vi "Single Slow IV v1.3.vi"() -> ()   [LabVIEW 2020]
uses:
  <vilib>/Utility/file.llb/Write Delimited Spreadsheet (DBL).vi
panel:
  in  "stop":bool
  in  "Tab Control 2":enum32{"cRIO plot", "Lockin X", "Lockin Y"}(tab)
  out "cRIO data plot":cluster{"Y":dbl[], "Y":dbl[]}[](graph)=[{"Y"=[0.1, 0.101, 0.10200000000000001, 0.10300000000000001, 0.10400000000000001, 0.10500000000000001, 0.10600000000000001, 0.10700000000000001, 0.10800000000000001, 0.10900000000000001, 0.11, 0.111, 0.112, 0.113, 0.114, 0.115, 0.116, 0.117, 0.11800000000000001, 0.11900000000000001, 0.12000000000000001, 0.12100000000000001, 0.122, 0.123, 0.124, 0.125, 0.126, 0.127, 0.128, 0.129, 0.13, 0.131, 0.132, 0.133, 0.134, 0.135, 0.136, 0.137, 0.138, 0.139, 0.14, 0.14100000000000001, 0.14200000000000002, 0.14300000000000002, 0.14400000000000002, 0.14500000000000002, 0.14600000000000002, 0.14700000000000002, 0.14800000000000002, 0.14900000000000002, 0.15000000000000002, 0.15100000000000002, 0.15200000000000002, 0.153, 0.154, 0.155, 0.156, 0.157, 0.158, 0.159, 0.16, 0.161, 0.162, 0.163, 0.164, 0.165, 0.166, 0.167, 0.168, 0.169, 0.17, 0.171, 0.17200000000000001, 0.173, 0.174, 0.175, 0.176, 0.177, 0.178, 0.179, 0.18, 0.181, 0.182, 0.183, 0.184, 0.185, 0.186, 0.187, 0.188, 0.189, 0.19, 0.191, 0.192, 0.193, 0.194, 0.195, 0.196, 0.197, 0.198, 0.199, 0.2], "Y"=[1.91443115234375e-05, 1.8234204101562503e-05, 1.8079296875e-05, 1.72965576171875e-05, 1.73908447265625e-05, 1.6982641601562502e-05, 1.7475024414062502e-05, 1.7350537109375e-05, 1.80681884765625e-05, 1.8036865234375e-05, 1.8520703124999998e-05, 1.9111669921875e-05, 1.948046875e-05, 1.9645117187500002e-05, 1.95529296875e-05, 1.9983398437500002e-05, 1.99129638671875e-05, 1.99599365234375e-05, 1.8666650390625e-05, 1.8764892578125e-05, 1.78889892578125e-05, 1.7660498046875002e-05, 1.7441210937500002e-05, 1.69652587890625e-05, 1.67341064453125e-05, 1.5950341796875e-05, 1.6491918945312503e-05, 1.61111572265625e-05, 1.6419482421875e-05, 1.6167163085937502e-05, 1.6684667968750002e-05, 1.66596923828125e-05, 1.76610595703125e-05, 1.7373608398437503e-05, 1.7419580078125e-05, 1.7511450195312502e-05, 1.76984619140625e-05, 1.7275e-05, 1.8423168945312502e-05, 1.78859619140625e-05, 1.74806396484375e-05, 1.7222802734375003e-05, 1.6946435546875e-05, 1.5935034179687498e-05, 1.5810864257812502e-05, 1.527841796875e-05, 1.509169921875e-05, 1.4530908203125001e-05, 1.4473876953125001e-05, 1.4885107421875e-05, 1.4928662109374999e-05, 1.5158349609375e-05, 1.5753149414062502e-05, 1.6247314453125003e-05, 1.59515625e-05, 1.62923583984375e-05, 1.64744873046875e-05, 1.65873779296875e-05, 1.7040673828125e-05, 1.65896484375e-05, 1.76021484375e-05, 1.6583422851562498e-05, 1.6492236328125e-05, 1.5975390625e-05, 1.57067138671875e-05, 1.4773681640625001e-05, 1.5178466796875001e-05, 1.4151171875e-05, 1.4718139648437501e-05, 1.453740234375e-05, 1.45205322265625e-05, 1.39417724609375e-05, 1.42656982421875e-05, 1.4501342773437501e-05, 1.4439892578125e-05, 1.47739501953125e-05, 1.47328369140625e-05, 1.46720703125e-05, 1.51514404296875e-05, 1.5362841796875e-05, 1.5647558593750002e-05, 1.612255859375e-05, 1.57461181640625e-05, 1.56584716796875e-05, 1.5264282226562502e-05, 1.4975024414062499e-05, 1.4608837890625003e-05, 1.4593286132812501e-05, 1.44783935546875e-05, 1.40139404296875e-05, 1.36931640625e-05, 1.3610986328125e-05, 1.3888769531250001e-05, 1.35940673828125e-05, 1.35070068359375e-05, 1.3863745117187502e-05, 1.45044677734375e-05, 1.418330078125e-05, 1.45068115234375e-05, 1.4514819335937501e-05, 1.4418505859375001e-05]}, {"Y"=[0.1, 0.101, 0.10200000000000001, 0.10300000000000001, 0.10400000000000001, 0.10500000000000001, 0.10600000000000001, 0.10700000000000001, 0.10800000000000001, 0.10900000000000001, 0.11, 0.111, 0.112, 0.113, 0.114, 0.115, 0.116, 0.117, 0.11800000000000001, 0.11900000000000001, 0.12000000000000001, 0.12100000000000001, 0.122, 0.123, 0.124, 0.125, 0.126, 0.127, 0.128, 0.129, 0.13, 0.131, 0.132, 0.133, 0.134, 0.135, 0.136, 0.137, 0.138, 0.139, 0.14, 0.14100000000000001, 0.14200000000000002, 0.14300000000000002, 0.14400000000000002, 0.14500000000000002, 0.14600000000000002, 0.14700000000000002, 0.14800000000000002, 0.14900000000000002, 0.15000000000000002, 0.15100000000000002, 0.15200000000000002, 0.153, 0.154, 0.155, 0.156, 0.157, 0.158, 0.159, 0.16, 0.161, 0.162, 0.163, 0.164, 0.165, 0.166, 0.167, 0.168, 0.169, 0.17, 0.171, 0.17200000000000001, 0.173, 0.174, 0.175, 0.176, 0.177, 0.178, 0.179, 0.18, 0.181, 0.182, 0.183, 0.184, 0.185, 0.186, 0.187, 0.188, 0.189, 0.19, 0.191, 0.192, 0.193, 0.194, 0.195, 0.196, 0.197, 0.198, 0.199, 0.2], "Y"=[2.07511962890625, 2.0750732421875, 2.074141357421875, 2.075462646484375, 2.075708740234375, 2.074308349609375, 2.074795654296875, 2.07555810546875, 2.0755185546875, 2.07468310546875, 2.074645751953125, 2.074962646484375, 2.0738427734375, 2.074322509765625, 2.07427294921875, 2.074574951171875, 2.075367431640625, 2.07494384765625, 2.074665771484375, 2.074663330078125, 2.07564013671875, 2.074562255859375, 2.074658935546875, 2.074733154296875, 2.07546826171875, 2.074733154296875, 2.074750244140625, 2.07523779296875, 2.07525244140625, 2.074369384765625, 2.075072265625, 2.0747587890625, 2.075584228515625, 2.075943603515625, 2.074529541015625, 2.07461474609375, 2.075067138671875, 2.075061279296875, 2.07536279296875, 2.07553466796875, 2.074748779296875, 2.075227294921875, 2.074936279296875, 2.075556396484375, 2.0753974609375, 2.0758994140625, 2.0761806640625, 2.075328369140625, 2.07436767578125, 2.076673828125, 2.076259765625, 2.075400146484375, 2.075468505859375, 2.075495849609375, 2.076040283203125, 2.0754658203125, 2.075578125, 2.0752451171875, 2.07488134765625, 2.07554736328125, 2.0753955078125, 2.0752822265625, 2.075176513671875, 2.076365478515625, 2.076373046875, 2.076056884765625, 2.07583837890625, 2.075223388671875, 2.0750703125, 2.07514599609375, 2.075769775390625, 2.0751220703125, 2.07619775390625, 2.075202392578125, 2.075671630859375, 2.07513916015625, 2.076079345703125, 2.076094970703125, 2.075864501953125, 2.07488134765625, 2.07613525390625, 2.076350341796875, 2.07625, 2.07523876953125, 2.075680419921875, 2.0746162109375, 2.076003173828125, 2.0753193359375, 2.075281494140625, 2.0755927734375, 2.075462158203125, 2.07468505859375, 2.07553564453125, 2.075280517578125, 2.0758173828125, 2.075341796875, 2.07434033203125, 2.074906005859375, 2.074229248046875, 2.0753671875, 2.0744853515625]}, {"Y"=[0.1, 0.101, 0.10200000000000001, 0.10300000000000001, 0.10400000000000001, 0.10500000000000001, 0.10600000000000001, 0.10700000000000001, 0.10800000000000001, 0.10900000000000001, 0.11, 0.111, 0.112, 0.113, 0.114, 0.115, 0.116, 0.117, 0.11800000000000001, 0.11900000000000001, 0.12000000000000001, 0.12100000000000001, 0.122, 0.123, 0.124, 0.125, 0.126, 0.127, 0.128, 0.129, 0.13, 0.131, 0.132, 0.133, 0.134, 0.135, 0.136, 0.137, 0.138, 0.139, 0.14, 0.14100000000000001, 0.14200000000000002, 0.14300000000000002, 0.14400000000000002, 0.14500000000000002, 0.14600000000000002, 0.14700000000000002, 0.14800000000000002, 0.14900000000000002, 0.15000000000000002, 0.15100000000000002, 0.15200000000000002, 0.153, 0.154, 0.155, 0.156, 0.157, 0.158, 0.159, 0.16, 0.161, 0.162, 0.163, 0.164, 0.165, 0.166, 0.167, 0.168, 0.169, 0.17, 0.171, 0.17200000000000001, 0.173, 0.174, 0.175, 0.176, 0.177, 0.178, 0.179, 0.18, 0.181, 0.182, 0.183, 0.184, 0.185, 0.186, 0.187, 0.188, 0.189, 0.19, 0.191, 0.192, 0.193, 0.194, 0.195, 0.196, 0.197, 0.198, 0.199, 0.2], "Y"=[0.000849365234375, 0.0008095703125, 0.000814453125, 0.00078076171875, 0.000771240234375, 0.000831787109375, 0.000755859375, 0.00079150390625, 0.0008310546875, 0.00079150390625, 0.00074560546875, 0.00078369140625, 0.000753662109375, 0.00079296875, 0.0007275390625, 0.000805419921875, 0.00074658203125, 0.00084375, 0.000741943359375, 0.00080859375, 0.00072705078125, 0.0007802734375, 0.0007021484375, 0.0008046875, 0.000873779296875, 0.000772216796875, 0.0007861328125, 0.000777587890625, 0.00078466796875, 0.00077001953125, 0.000764404296875, 0.0007626953125, 0.000732421875, 0.00077783203125, 0.00079150390625, 0.0007861328125, 0.000770751953125, 0.0008134765625, 0.00080419921875, 0.00079345703125, 0.000803466796875, 0.0007470703125, 0.000757080078125, 0.000783935546875, 0.000799072265625, 0.000781982421875, 0.00076904296875, 0.000742919921875, 0.00082666015625, 0.00078369140625, 0.000858154296875, 0.00076318359375, 0.0006982421875, 0.00071728515625, 0.00077099609375, 0.00078076171875, 0.000766845703125, 0.00076806640625, 0.000752197265625, 0.000720703125, 0.00075830078125, 0.00077099609375, 0.0008076171875, 0.000795166015625, 0.00074365234375, 0.000795166015625, 0.00078125, 0.000791748046875, 0.000809814453125, 0.00074755859375, 0.000774658203125, 0.000756103515625, 0.00083251953125, 0.000758056640625, 0.00082470703125, 0.00077197265625, 0.000834228515625, 0.000770751953125, 0.00077734375, 0.000760009765625, 0.000823974609375, 0.00071533203125, 0.000766357421875, 0.0007548828125, 0.000796630859375, 0.000743408203125, 0.000770751953125, 0.000744384765625, 0.0007314453125, 0.000734130859375, 0.000804443359375, 0.0007275390625, 0.000815673828125, 0.000766357421875, 0.000784912109375, 0.000762451171875, 0.00075, 0.000779296875, 0.000757080078125, 0.000751953125, 0.000764892578125]}, {"Y"=[0.1, 0.101, 0.10200000000000001, 0.10300000000000001, 0.10400000000000001, 0.10500000000000001, 0.10600000000000001, 0.10700000000000001, 0.10800000000000001, 0.10900000000000001, 0.11, 0.111, 0.112, 0.113, 0.114, 0.115, 0.116, 0.117, 0.11800000000000001, 0.11900000000000001, 0.12000000000000001, 0.12100000000000001, 0.122, 0.123, 0.124, 0.125, 0.126, 0.127, 0.128, 0.129, 0.13, 0.131, 0.132, 0.133, 0.134, 0.135, 0.136, 0.137, 0.138, 0.139, 0.14, 0.14100000000000001, 0.14200000000000002, 0.14300000000000002, 0.14400000000000002, 0.14500000000000002, 0.14600000000000002, 0.14700000000000002, 0.14800000000000002, 0.14900000000000002, 0.15000000000000002, 0.15100000000000002, 0.15200000000000002, 0.153, 0.154, 0.155, 0.156, 0.157, 0.158, 0.159, 0.16, 0.161, 0.162, 0.163, 0.164, 0.165, 0.166, 0.167, 0.168, 0.169, 0.17, 0.171, 0.17200000000000001, 0.173, 0.174, 0.175, 0.176, 0.177, 0.178, 0.179, 0.18, 0.181, 0.182, 0.183, 0.184, 0.185, 0.186, 0.187, 0.188, 0.189, 0.19, 0.191, 0.192, 0.193, 0.194, 0.195, 0.196, 0.197, 0.198, 0.199, 0.2], "Y"=[0.00172021484375, 0.001699462890625, 0.001721435546875, 0.001740966796875, 0.001722412109375, 0.001780517578125, 0.001792724609375, 0.00180224609375, 0.001711181640625, 0.00181494140625, 0.001773193359375, 0.001771240234375, 0.00173388671875, 0.001708740234375, 0.00180908203125, 0.001841064453125, 0.001756103515625, 0.00170068359375, 0.00175, 0.001714111328125, 0.001801025390625, 0.001765625, 0.0017099609375, 0.001703857421875, 0.001786865234375, 0.0018046875, 0.001700927734375, 0.001765380859375, 0.001693603515625, 0.00175244140625, 0.0017626953125, 0.0017978515625, 0.001715576171875, 0.001716064453125, 0.00177099609375, 0.00180712890625, 0.001722900390625, 0.001816650390625, 0.001749755859375, 0.00174755859375, 0.001776123046875, 0.00170849609375, 0.00172509765625, 0.001736083984375, 0.00171533203125, 0.001705322265625, 0.001744873046875, 0.001779296875, 0.001696044921875, 0.00173974609375, 0.001815185546875, 0.001720947265625, 0.00178076171875, 0.001763916015625, 0.0017958984375, 0.0017158203125, 0.00179248046875, 0.001754638671875, 0.00173193359375, 0.001706298828125, 0.00173388671875, 0.00166943359375, 0.0017373046875, 0.001741943359375, 0.001747314453125, 0.001755615234375, 0.001791748046875, 0.001772216796875, 0.001737548828125, 0.00176904296875, 0.00175830078125, 0.001655029296875, 0.001769775390625, 0.001682861328125, 0.00176318359375, 0.00177294921875, 0.00177001953125, 0.00178271484375, 0.00175537109375, 0.00174755859375, 0.001724365234375, 0.001774658203125, 0.0017412109375, 0.001767333984375, 0.00175341796875, 0.0017685546875, 0.0017138671875, 0.0017158203125, 0.00172998046875, 0.001653076171875, 0.0017529296875, 0.001751708984375, 0.001750244140625, 0.00172265625, 0.00180859375, 0.00176953125, 0.00177490234375, 0.001733154296875, 0.001750244140625, 0.001706298828125, 0.0017529296875]}]
  out "cRIO Plot 0":string="DC Voltage V"
  out "cRIO Plot 1":string="DC current uA"
  out "cRIO Plot 2":string="dV V"
  out "cRIO Plot 3":string="dI uA"
  out "Lockin X":cluster{"Y":dbl[], "Y":dbl[]}[](graph)=[{"Y"=[0.1, 0.101, 0.10200000000000001, 0.10300000000000001, 0.10400000000000001, 0.10500000000000001, 0.10600000000000001, 0.10700000000000001, 0.10800000000000001, 0.10900000000000001, 0.11, 0.111, 0.112, 0.113, 0.114, 0.115, 0.116, 0.117, 0.11800000000000001, 0.11900000000000001, 0.12000000000000001, 0.12100000000000001, 0.122, 0.123, 0.124, 0.125, 0.126, 0.127, 0.128, 0.129, 0.13, 0.131, 0.132, 0.133, 0.134, 0.135, 0.136, 0.137, 0.138, 0.139, 0.14, 0.14100000000000001, 0.14200000000000002, 0.14300000000000002, 0.14400000000000002, 0.14500000000000002, 0.14600000000000002, 0.14700000000000002, 0.14800000000000002, 0.14900000000000002, 0.15000000000000002, 0.15100000000000002, 0.15200000000000002, 0.153, 0.154, 0.155, 0.156, 0.157, 0.158, 0.159, 0.16, 0.161, 0.162, 0.163, 0.164, 0.165, 0.166, 0.167, 0.168, 0.169, 0.17, 0.171, 0.17200000000000001, 0.173, 0.174, 0.175, 0.176, 0.177, 0.178, 0.179, 0.18, 0.181, 0.182, 0.183, 0.184, 0.185, 0.186, 0.187, 0.188, 0.189, 0.19, 0.191, 0.192, 0.193, 0.194, 0.195, 0.196, 0.197, 0.198, 0.199, 0.2], "Y"=[1.41335, 1.26267, 0.92316, 1.13488, 1.13869, 1.297, 1.30273, 1.3466, 1.35041, 1.09673, 1.13679, 1.0013699999999999, 1.02998, 1.0681200000000002, 0.974659, 0.8926430000000001, 1.33706, 1.05477, 1.02235, 1.29319, 1.03951, 1.3141699999999998, 1.31989, 1.35613, 1.07766, 0.74387, 0.795368, 0.93079, 0.812534, 0.8869210000000001, 1.02235, 1.12153, 1.23788, 1.0585900000000001, 1.02807, 0.928883, 1.13488, 0.9727520000000001, 0.86594, 0.856403, 0.812534, 0.8754770000000001, 1.0604900000000002, 0.963215, 0.957493, 1.00899, 1.08147, 0.8697550000000001, 0.974659, 1.14632, 1.0585900000000001, 0.963215, 0.633243, 0.770573, 1.03761, 0.911716, 0.9594, 1.08529, 1.10436, 1.07766, 0.822071, 0.879291, 1.11008, 1.17493, 1.05477, 0.909809, 0.720982, 0.629429, 0.698093, 0.909809, 0.967029, 0.913624, 0.92316, 0.810627, 0.949863, 1.07384, 1.14823, 1.22262, 1.0662200000000002, 1.01281, 0.8697550000000001, 1.0604900000000002, 0.9594, 0.734333, 0.8316079999999999, 0.835422, 0.8964580000000001, 0.764851, 0.804905, 0.791553, 0.947956, 0.5817450000000001, 0.654224, 0.625614, 0.631336, 0.711445, 0.730518, 0.606541, 0.633243, 0.703815, 0.646595]}, {"Y"=[0.1, 0.101, 0.10200000000000001, 0.10300000000000001, 0.10400000000000001, 0.10500000000000001, 0.10600000000000001, 0.10700000000000001, 0.10800000000000001, 0.10900000000000001, 0.11, 0.111, 0.112, 0.113, 0.114, 0.115, 0.116, 0.117, 0.11800000000000001, 0.11900000000000001, 0.12000000000000001, 0.12100000000000001, 0.122, 0.123, 0.124, 0.125, 0.126, 0.127, 0.128, 0.129, 0.13, 0.131, 0.132, 0.133, 0.134, 0.135, 0.136, 0.137, 0.138, 0.139, 0.14, 0.14100000000000001, 0.14200000000000002, 0.14300000000000002, 0.14400000000000002, 0.14500000000000002, 0.14600000000000002, 0.14700000000000002, 0.14800000000000002, 0.14900000000000002, 0.15000000000000002, 0.15100000000000002, 0.15200000000000002, 0.153, 0.154, 0.155, 0.156, 0.157, 0.158, 0.159, 0.16, 0.161, 0.162, 0.163, 0.164, 0.165, 0.166, 0.167, 0.168, 0.169, 0.17, 0.171, 0.17200000000000001, 0.173, 0.174, 0.175, 0.176, 0.177, 0.178, 0.179, 0.18, 0.181, 0.182, 0.183, 0.184, 0.185, 0.186, 0.187, 0.188, 0.189, 0.19, 0.191, 0.192, 0.193, 0.194, 0.195, 0.196, 0.197, 0.198, 0.199, 0.2], "Y"=[0.755314, 0.915531, 0.9594, 0.967029, 0.9727520000000001, 0.970844, 0.970844, 0.974659, 0.970844, 0.974659, 0.974659, 0.974659, 0.9727520000000001, 0.9727520000000001, 0.974659, 0.970844, 0.9727520000000001, 0.9765699999999999, 0.9765699999999999, 0.9765699999999999, 0.974659, 0.9765699999999999, 0.9803850000000001, 0.9765699999999999, 0.9765699999999999, 0.974659, 0.9727520000000001, 0.9727520000000001, 0.9727520000000001, 0.9765699999999999, 0.974659, 0.9784769999999999, 0.9784769999999999, 0.974659, 0.968937, 0.967029, 0.970844, 0.9765699999999999, 0.9765699999999999, 0.974659, 0.9727520000000001, 0.9727520000000001, 0.9765699999999999, 0.9765699999999999, 0.9765699999999999, 0.974659, 0.9765699999999999, 0.9765699999999999, 0.9765699999999999, 0.9727520000000001, 0.9727520000000001, 0.9765699999999999, 0.9803850000000001, 0.982292, 0.9784769999999999, 0.9784769999999999, 0.974659, 0.974659, 0.9765699999999999, 0.974659, 0.974659, 0.9727520000000001, 0.9765699999999999, 0.9784769999999999, 0.984199, 0.982292, 0.9765699999999999, 0.9765699999999999, 0.974659, 0.974659, 0.9765699999999999, 0.9765699999999999, 0.9765699999999999, 0.9784769999999999, 0.9765699999999999, 0.9765699999999999, 0.9765699999999999, 0.9765699999999999, 0.974659, 0.9765699999999999, 0.9765699999999999, 0.9765699999999999, 0.970844, 0.970844, 0.9765699999999999, 0.9727520000000001, 0.970844, 0.968937, 0.9727520000000001, 0.9765699999999999, 0.9765699999999999, 0.9784769999999999, 0.9765699999999999, 0.9765699999999999, 0.9765699999999999, 0.9765699999999999, 0.9727520000000001, 0.968937, 0.968937, 0.967029, 0.9727520000000001]}, {"Y"=[0.1, 0.101, 0.10200000000000001, 0.10300000000000001, 0.10400000000000001, 0.10500000000000001, 0.10600000000000001, 0.10700000000000001, 0.10800000000000001, 0.10900000000000001, 0.11, 0.111, 0.112, 0.113, 0.114, 0.115, 0.116, 0.117, 0.11800000000000001, 0.11900000000000001, 0.12000000000000001, 0.12100000000000001, 0.122, 0.123, 0.124, 0.125, 0.126, 0.127, 0.128, 0.129, 0.13, 0.131, 0.132, 0.133, 0.134, 0.135, 0.136, 0.137, 0.138, 0.139, 0.14, 0.14100000000000001, 0.14200000000000002, 0.14300000000000002, 0.14400000000000002, 0.14500000000000002, 0.14600000000000002, 0.14700000000000002, 0.14800000000000002, 0.14900000000000002, 0.15000000000000002, 0.15100000000000002, 0.15200000000000002, 0.153, 0.154, 0.155, 0.156, 0.157, 0.158, 0.159, 0.16, 0.161, 0.162, 0.163, 0.164, 0.165, 0.166, 0.167, 0.168, 0.169, 0.17, 0.171, 0.17200000000000001, 0.173, 0.174, 0.175, 0.176, 0.177, 0.178, 0.179, 0.18, 0.181, 0.182, 0.183, 0.184, 0.185, 0.186, 0.187, 0.188, 0.189, 0.19, 0.191, 0.192, 0.193, 0.194, 0.195, 0.196, 0.197, 0.198, 0.199, 0.2], "Y"=[0.0, 0.0, 0.0, 0.0, 0.0, 0.0, 0.0, 0.0, 0.0, 0.0, 0.0, 0.0, 0.0, 0.0, 0.0, 0.0, 0.0, 0.0, 0.0, 0.0, 0.0, 0.0, 0.0, 0.0, 0.0, 0.0, 0.0, 0.0, 0.0, 0.0, 0.0, 0.0, 0.0, 0.0, 0.0, 0.0, 0.0, 0.0, 0.0, 0.0, 0.0, 0.0, 0.0, 0.0, 0.0, 0.0, 0.0, 0.0, 0.0, 0.0, 0.0, 0.0, 0.0, 0.0, 0.0, 0.0, 0.0, 0.0, 0.0, 0.0, 0.0, 0.0, 0.0, 0.0, 0.0, 0.0, 0.0, 0.0, 0.0, 0.0, 0.0, 0.0, 0.0, 0.0, 0.0, 0.0, 0.0, 0.0, 0.0, 0.0, 0.0, 0.0, 0.0, 0.0, 0.0, 0.0, 0.0, 0.0, 0.0, 0.0, 0.0, 0.0, 0.0, 0.0, 0.0, 0.0, 0.0, 0.0, 0.0, 0.0, 0.0]}, {"Y"=[0.1, 0.101, 0.10200000000000001, 0.10300000000000001, 0.10400000000000001, 0.10500000000000001, 0.10600000000000001, 0.10700000000000001, 0.10800000000000001, 0.10900000000000001, 0.11, 0.111, 0.112, 0.113, 0.114, 0.115, 0.116, 0.117, 0.11800000000000001, 0.11900000000000001, 0.12000000000000001, 0.12100000000000001, 0.122, 0.123, 0.124, 0.125, 0.126, 0.127, 0.128, 0.129, 0.13, 0.131, 0.132, 0.133, 0.134, 0.135, 0.136, 0.137, 0.138, 0.139, 0.14, 0.14100000000000001, 0.14200000000000002, 0.14300000000000002, 0.14400000000000002, 0.14500000000000002, 0.14600000000000002, 0.14700000000000002, 0.14800000000000002, 0.14900000000000002, 0.15000000000000002, 0.15100000000000002, 0.15200000000000002, 0.153, 0.154, 0.155, 0.156, 0.157, 0.158, 0.159, 0.16, 0.161, 0.162, 0.163, 0.164, 0.165, 0.166, 0.167, 0.168, 0.169, 0.17, 0.171, 0.17200000000000001, 0.173, 0.174, 0.175, 0.176, 0.177, 0.178, 0.179, 0.18, 0.181, 0.182, 0.183, 0.184, 0.185, 0.186, 0.187, 0.188, 0.189, 0.19, 0.191, 0.192, 0.193, 0.194, 0.195, 0.196, 0.197, 0.198, 0.199, 0.2], "Y"=[0.0, 0.0, 0.0, 0.0, 0.0, 0.0, 0.0, 0.0, 0.0, 0.0, 0.0, 0.0, 0.0, 0.0, 0.0, 0.0, 0.0, 0.0, 0.0, 0.0, 0.0, 0.0, 0.0, 0.0, 0.0, 0.0, 0.0, 0.0, 0.0, 0.0, 0.0, 0.0, 0.0, 0.0, 0.0, 0.0, 0.0, 0.0, 0.0, 0.0, 0.0, 0.0, 0.0, 0.0, 0.0, 0.0, 0.0, 0.0, 0.0, 0.0, 0.0, 0.0, 0.0, 0.0, 0.0, 0.0, 0.0, 0.0, 0.0, 0.0, 0.0, 0.0, 0.0, 0.0, 0.0, 0.0, 0.0, 0.0, 0.0, 0.0, 0.0, 0.0, 0.0, 0.0, 0.0, 0.0, 0.0, 0.0, 0.0, 0.0, 0.0, 0.0, 0.0, 0.0, 0.0, 0.0, 0.0, 0.0, 0.0, 0.0, 0.0, 0.0, 0.0, 0.0, 0.0, 0.0, 0.0, 0.0, 0.0, 0.0, 0.0]}]
  out "Lockin Y":cluster{"Y":dbl[], "Y":dbl[]}[](graph)=[{"Y"=[0.1, 0.101, 0.10200000000000001, 0.10300000000000001, 0.10400000000000001, 0.10500000000000001, 0.10600000000000001, 0.10700000000000001, 0.10800000000000001, 0.10900000000000001, 0.11, 0.111, 0.112, 0.113, 0.114, 0.115, 0.116, 0.117, 0.11800000000000001, 0.11900000000000001, 0.12000000000000001, 0.12100000000000001, 0.122, 0.123, 0.124, 0.125, 0.126, 0.127, 0.128, 0.129, 0.13, 0.131, 0.132, 0.133, 0.134, 0.135, 0.136, 0.137, 0.138, 0.139, 0.14, 0.14100000000000001, 0.14200000000000002, 0.14300000000000002, 0.14400000000000002, 0.14500000000000002, 0.14600000000000002, 0.14700000000000002, 0.14800000000000002, 0.14900000000000002, 0.15000000000000002, 0.15100000000000002, 0.15200000000000002, 0.153, 0.154, 0.155, 0.156, 0.157, 0.158, 0.159, 0.16, 0.161, 0.162, 0.163, 0.164, 0.165, 0.166, 0.167, 0.168, 0.169, 0.17, 0.171, 0.17200000000000001, 0.173, 0.174, 0.175, 0.176, 0.177, 0.178, 0.179, 0.18, 0.181, 0.182, 0.183, 0.184, 0.185, 0.186, 0.187, 0.188, 0.189, 0.19, 0.191, 0.192, 0.193, 0.194, 0.195, 0.196, 0.197, 0.198, 0.199, 0.2], "Y"=[-0.349047, -0.234605, -0.135423, -0.265123, -0.20408700000000002, -0.144959, -0.106812, 0.0953679, -0.0953679, -0.5397829999999999, -0.608448, -0.364305, -0.33951000000000003, -0.38337899999999997, -0.261309, -0.08010909999999999, 0.0114442, -0.0877385, 0.164033, 0.0381472, -0.034332499999999995, -0.265123, -0.0915532, -0.026703, -0.0953679, -0.06866499999999999, -0.17357, -0.27275299999999997, -0.270845, -0.17357, -0.0762944, -0.23842000000000002, -0.253679, -0.175477, -0.316622, 0.0839238, -0.0743871, -0.278475, -0.164033, -0.23079, -0.305178, -0.33188100000000004, -0.234605, -0.16975500000000002, -0.278475, -0.146867, -0.186921, -0.389101, -0.411989, -0.349047, -0.20790199999999998, -0.026703, -0.26893799999999995, -0.13732999999999998, 0.0743871, -0.020981, -0.0667577, -0.156404, -0.167848, 0.110627, 0.400545, 0.16975500000000002, -0.118256, -0.034332499999999995, 0.108719, 0.167848, 0.127793, 0.07247970000000001, 0.062943, 0.0915532, 0.0839238, -0.0171663, 0.0572207, 0.053406, -0.23079, -0.16594, -0.307085, -0.379564, -0.118256, -0.125886, -0.183106, -0.125886, 0.0419619, -0.0667577, -0.055313299999999996, -0.059128, 0.034332499999999995, 0.0610356, -0.116349, -0.144959, -0.24605, -0.240327, -0.318529, -0.352861, -0.356676, -0.110627, -0.102997, -0.0972752, 0.20408700000000002, 0.144959, 0.20218]}, {"Y"=[0.1, 0.101, 0.10200000000000001, 0.10300000000000001, 0.10400000000000001, 0.10500000000000001, 0.10600000000000001, 0.10700000000000001, 0.10800000000000001, 0.10900000000000001, 0.11, 0.111, 0.112, 0.113, 0.114, 0.115, 0.116, 0.117, 0.11800000000000001, 0.11900000000000001, 0.12000000000000001, 0.12100000000000001, 0.122, 0.123, 0.124, 0.125, 0.126, 0.127, 0.128, 0.129, 0.13, 0.131, 0.132, 0.133, 0.134, 0.135, 0.136, 0.137, 0.138, 0.139, 0.14, 0.14100000000000001, 0.14200000000000002, 0.14300000000000002, 0.14400000000000002, 0.14500000000000002, 0.14600000000000002, 0.14700000000000002, 0.14800000000000002, 0.14900000000000002, 0.15000000000000002, 0.15100000000000002, 0.15200000000000002, 0.153, 0.154, 0.155, 0.156, 0.157, 0.158, 0.159, 0.16, 0.161, 0.162, 0.163, 0.164, 0.165, 0.166, 0.167, 0.168, 0.169, 0.17, 0.171, 0.17200000000000001, 0.173, 0.174, 0.175, 0.176, 0.177, 0.178, 0.179, 0.18, 0.181, 0.182, 0.183, 0.184, 0.185, 0.186, 0.187, 0.188, 0.189, 0.19, 0.191, 0.192, 0.193, 0.194, 0.195, 0.196, 0.197, 0.198, 0.199, 0.2], "Y"=[-0.20790199999999998, -0.114441, -0.0915532, -0.0858312, -0.08010909999999999, -0.0820165, -0.0858312, -0.0839238, -0.0858312, -0.0858312, -0.0858312, -0.0896459, -0.0839238, -0.0858312, -0.0858312, -0.0877385, -0.0877385, -0.0839238, -0.0820165, -0.0858312, -0.0820165, -0.0839238, -0.0858312, -0.0896459, -0.0915532, -0.0877385, -0.0839238, -0.0877385, -0.0877385, -0.0820165, -0.0839238, -0.0820165, -0.0839238, -0.0839238, -0.08010909999999999, -0.0839238, -0.0820165, -0.0877385, -0.0839238, -0.0858312, -0.0858312, -0.0820165, -0.0820165, -0.08010909999999999, -0.0877385, -0.0915532, -0.0934605, -0.0877385, -0.0820165, -0.08010909999999999, -0.08010909999999999, -0.0858312, -0.0820165, -0.0820165, -0.0896459, -0.0877385, -0.0877385, -0.0858312, -0.0839238, -0.08010909999999999, -0.0858312, -0.0839238, -0.08010909999999999, -0.08010909999999999, -0.0839238, -0.08010909999999999, -0.0839238, -0.0877385, -0.0915532, -0.0858312, -0.0839238, -0.0858312, -0.0896459, -0.0915532, -0.0877385, -0.0839238, -0.08010909999999999, -0.08010909999999999, -0.0820165, -0.0820165, -0.0839238, -0.08010909999999999, -0.0839238, -0.0858312, -0.0858312, -0.0915532, -0.0896459, -0.0820165, -0.07820179999999999, -0.08010909999999999, -0.0820165, -0.08010909999999999, -0.0762944, -0.0820165, -0.0820165, -0.0858312, -0.0820165, -0.08010909999999999, -0.0858312, -0.0896459, -0.0877385]}, {"Y"=[0.1, 0.101, 0.10200000000000001, 0.10300000000000001, 0.10400000000000001, 0.10500000000000001, 0.10600000000000001, 0.10700000000000001, 0.10800000000000001, 0.10900000000000001, 0.11, 0.111, 0.112, 0.113, 0.114, 0.115, 0.116, 0.117, 0.11800000000000001, 0.11900000000000001, 0.12000000000000001, 0.12100000000000001, 0.122, 0.123, 0.124, 0.125, 0.126, 0.127, 0.128, 0.129, 0.13, 0.131, 0.132, 0.133, 0.134, 0.135, 0.136, 0.137, 0.138, 0.139, 0.14, 0.14100000000000001, 0.14200000000000002, 0.14300000000000002, 0.14400000000000002, 0.14500000000000002, 0.14600000000000002, 0.14700000000000002, 0.14800000000000002, 0.14900000000000002, 0.15000000000000002, 0.15100000000000002, 0.15200000000000002, 0.153, 0.154, 0.155, 0.156, 0.157, 0.158, 0.159, 0.16, 0.161, 0.162, 0.163, 0.164, 0.165, 0.166, 0.167, 0.168, 0.169, 0.17, 0.171, 0.17200000000000001, 0.173, 0.174, 0.175, 0.176, 0.177, 0.178, 0.179, 0.18, 0.181, 0.182, 0.183, 0.184, 0.185, 0.186, 0.187, 0.188, 0.189, 0.19, 0.191, 0.192, 0.193, 0.194, 0.195, 0.196, 0.197, 0.198, 0.199, 0.2], "Y"=[0.0, 0.0, 0.0, 0.0, 0.0, 0.0, 0.0, 0.0, 0.0, 0.0, 0.0, 0.0, 0.0, 0.0, 0.0, 0.0, 0.0, 0.0, 0.0, 0.0, 0.0, 0.0, 0.0, 0.0, 0.0, 0.0, 0.0, 0.0, 0.0, 0.0, 0.0, 0.0, 0.0, 0.0, 0.0, 0.0, 0.0, 0.0, 0.0, 0.0, 0.0, 0.0, 0.0, 0.0, 0.0, 0.0, 0.0, 0.0, 0.0, 0.0, 0.0, 0.0, 0.0, 0.0, 0.0, 0.0, 0.0, 0.0, 0.0, 0.0, 0.0, 0.0, 0.0, 0.0, 0.0, 0.0, 0.0, 0.0, 0.0, 0.0, 0.0, 0.0, 0.0, 0.0, 0.0, 0.0, 0.0, 0.0, 0.0, 0.0, 0.0, 0.0, 0.0, 0.0, 0.0, 0.0, 0.0, 0.0, 0.0, 0.0, 0.0, 0.0, 0.0, 0.0, 0.0, 0.0, 0.0, 0.0, 0.0, 0.0, 0.0]}, {"Y"=[0.1, 0.101, 0.10200000000000001, 0.10300000000000001, 0.10400000000000001, 0.10500000000000001, 0.10600000000000001, 0.10700000000000001, 0.10800000000000001, 0.10900000000000001, 0.11, 0.111, 0.112, 0.113, 0.114, 0.115, 0.116, 0.117, 0.11800000000000001, 0.11900000000000001, 0.12000000000000001, 0.12100000000000001, 0.122, 0.123, 0.124, 0.125, 0.126, 0.127, 0.128, 0.129, 0.13, 0.131, 0.132, 0.133, 0.134, 0.135, 0.136, 0.137, 0.138, 0.139, 0.14, 0.14100000000000001, 0.14200000000000002, 0.14300000000000002, 0.14400000000000002, 0.14500000000000002, 0.14600000000000002, 0.14700000000000002, 0.14800000000000002, 0.14900000000000002, 0.15000000000000002, 0.15100000000000002, 0.15200000000000002, 0.153, 0.154, 0.155, 0.156, 0.157, 0.158, 0.159, 0.16, 0.161, 0.162, 0.163, 0.164, 0.165, 0.166, 0.167, 0.168, 0.169, 0.17, 0.171, 0.17200000000000001, 0.173, 0.174, 0.175, 0.176, 0.177, 0.178, 0.179, 0.18, 0.181, 0.182, 0.183, 0.184, 0.185, 0.186, 0.187, 0.188, 0.189, 0.19, 0.191, 0.192, 0.193, 0.194, 0.195, 0.196, 0.197, 0.198, 0.199, 0.2], "Y"=[0.0, 0.0, 0.0, 0.0, 0.0, 0.0, 0.0, 0.0, 0.0, 0.0, 0.0, 0.0, 0.0, 0.0, 0.0, 0.0, 0.0, 0.0, 0.0, 0.0, 0.0, 0.0, 0.0, 0.0, 0.0, 0.0, 0.0, 0.0, 0.0, 0.0, 0.0, 0.0, 0.0, 0.0, 0.0, 0.0, 0.0, 0.0, 0.0, 0.0, 0.0, 0.0, 0.0, 0.0, 0.0, 0.0, 0.0, 0.0, 0.0, 0.0, 0.0, 0.0, 0.0, 0.0, 0.0, 0.0, 0.0, 0.0, 0.0, 0.0, 0.0, 0.0, 0.0, 0.0, 0.0, 0.0, 0.0, 0.0, 0.0, 0.0, 0.0, 0.0, 0.0, 0.0, 0.0, 0.0, 0.0, 0.0, 0.0, 0.0, 0.0, 0.0, 0.0, 0.0, 0.0, 0.0, 0.0, 0.0, 0.0, 0.0, 0.0, 0.0, 0.0, 0.0, 0.0, 0.0, 0.0, 0.0, 0.0, 0.0, 0.0]}]
  in  "Tab Control":enum32{"cRIO", "variable", "Lockin", "Status"}(tab)=enum."variable"
  in  "cRIO Chan 0":bool=TRUE
  in  "cRIO IP":string="//172.22.11.2"
  in  "Reading Average times":i32=1000
  in  "read cRIO":bool=TRUE
  in  "Scale factor3":dbl=1.0
  in  "Channel name 3":string(combo)="dI uA"
  in  "cRIO Chan 3":bool
  in  "Scale factor2":dbl=1.0
  in  "Channel name 2":string(combo)="dV V"
  in  "cRIO Chan 2":bool
  in  "Scale factor1":dbl=1.0
  in  "Channel name 1":string(combo)="DC current uA"
  in  "cRIO Chan 1":bool=TRUE
  in  "Scale factor0":dbl=0.0001
  in  "Channel name 0":string(combo)="DC Voltage V"
  out "Unit":string="mT"
  in  "Tab for variable":enum32{"Current", "Magnetic field"}(tab)=enum."Magnetic field"
  in  "Delay Time s":dbl=1.5 caption="Delay Time (s)"
  in  "AO Channel":string(combo)="AO0"
  in  "current output Scale factor":dbl=1.0
  in  "Fixed current uA":dbl=2.1
  in  "Scale factor":dbl=1.0
  in  "Field Rate mT per sec":dbl=0.1 format="%#_13g"
  in  "Magnet Device Select":string(combo)="NI DAQ Controlled V to I source"
  in  "Start":dbl=0.1
  in  "Range":dbl=0.1
  in  "Step":dbl=0.001
  in  "Ramp type":string(combo)="Range"
  in  "Ramp up first T":bool=TRUE
  in  "Lockin address 4":string
  in  "Lockin address 3":string
  in  "Lockin address 2":string="GPIB0::9::INSTR"
  in  "Lockin address 1":string="GPIB0::8::INSTR"
  in  "Lockin 4":bool
  in  "Lockin 3":bool
  in  "Lockin 2":bool=TRUE
  in  "Lockin 1":bool=TRUE
  in  "Use Lockin":bool=TRUE
  in  "Lockin Chan name 4":string(combo)="None"
  in  "Lockin Chan name 3":string(combo)="None"
  in  "Lockin Chan name 2":string(combo)="Current mV"
  in  "Lockin Chan name 1":string(combo)="Voltage mV"
  in  "Lockin and field and temperature status":string="Data File time stamp 20210723-212111\nTemperature Chan1 1.218210, Chan2 0.050013\nmagnetic field InfmT\nLockin status\n#Device channel name Voltage mV#Device \u0000\u0000\u0000\u000fGPIB0::8::INSTR\n #PHASE=0\n #REF=1\n #FREQ=17\n #INPUT=0\n #SENS=22\n #TIMECONST=10\n #VOLTAGE=0.1\n#Device channel name Current mV#Device \u0000\u0000\u0000\u000fGPIB0::9::INSTR\n #PHASE=0\n #REF=0\n #FREQ=16.9997\n #INPUT=0\n #SENS=22\n #TIMECONST=10\n #VOLTAGE=0.004\n"
  in  "Temp Device":string(combo)="Elsa"
  in  "Temp Chan1":string="T5"
  in  "Temp Chan2":string="T8"
  in  "Magnetic field read device":string(combo)="Elsa Magnet"
  in  "Record Field":bool
  in  "Contour plot folder":path=path "C:/Users/gyue/Desktop/Data folder 20210720"
  out "error out":errorcluster
  # "Voltage x factor=actual"
  # "Voltage x factor=uA"
  # "Voltage x factor=uA"
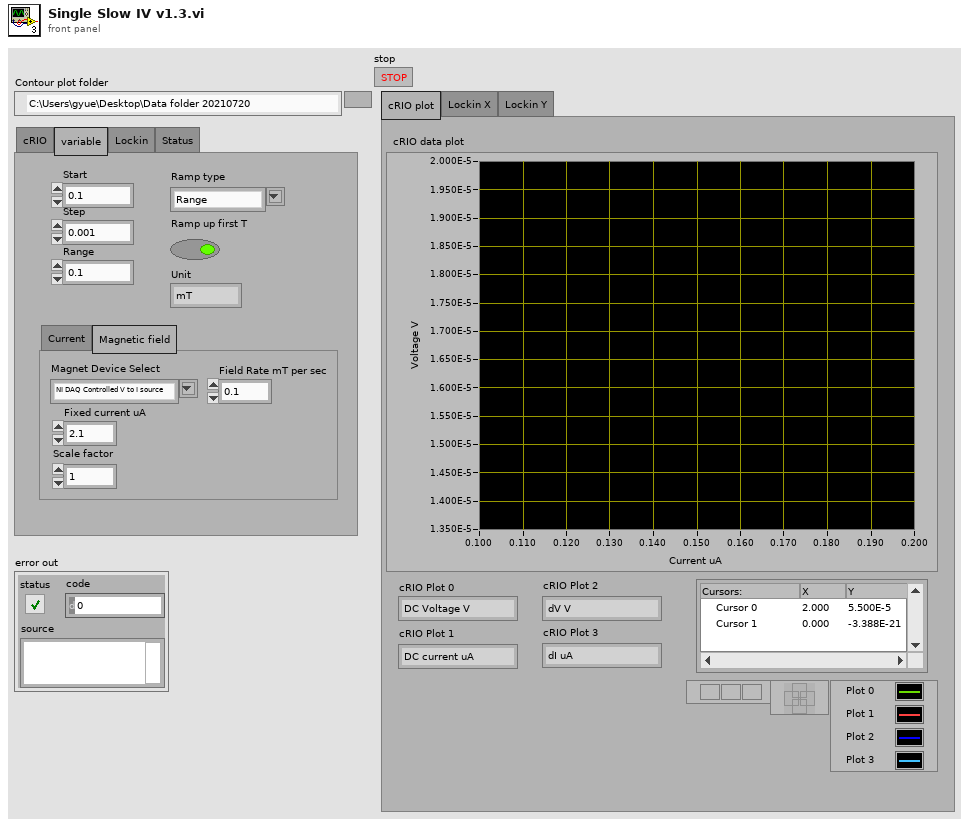
[diagram p1: front panel]
types:
  T1 = cluster{"AI0":dbl, "AI1":dbl, "AI2":dbl, "AI3":dbl}
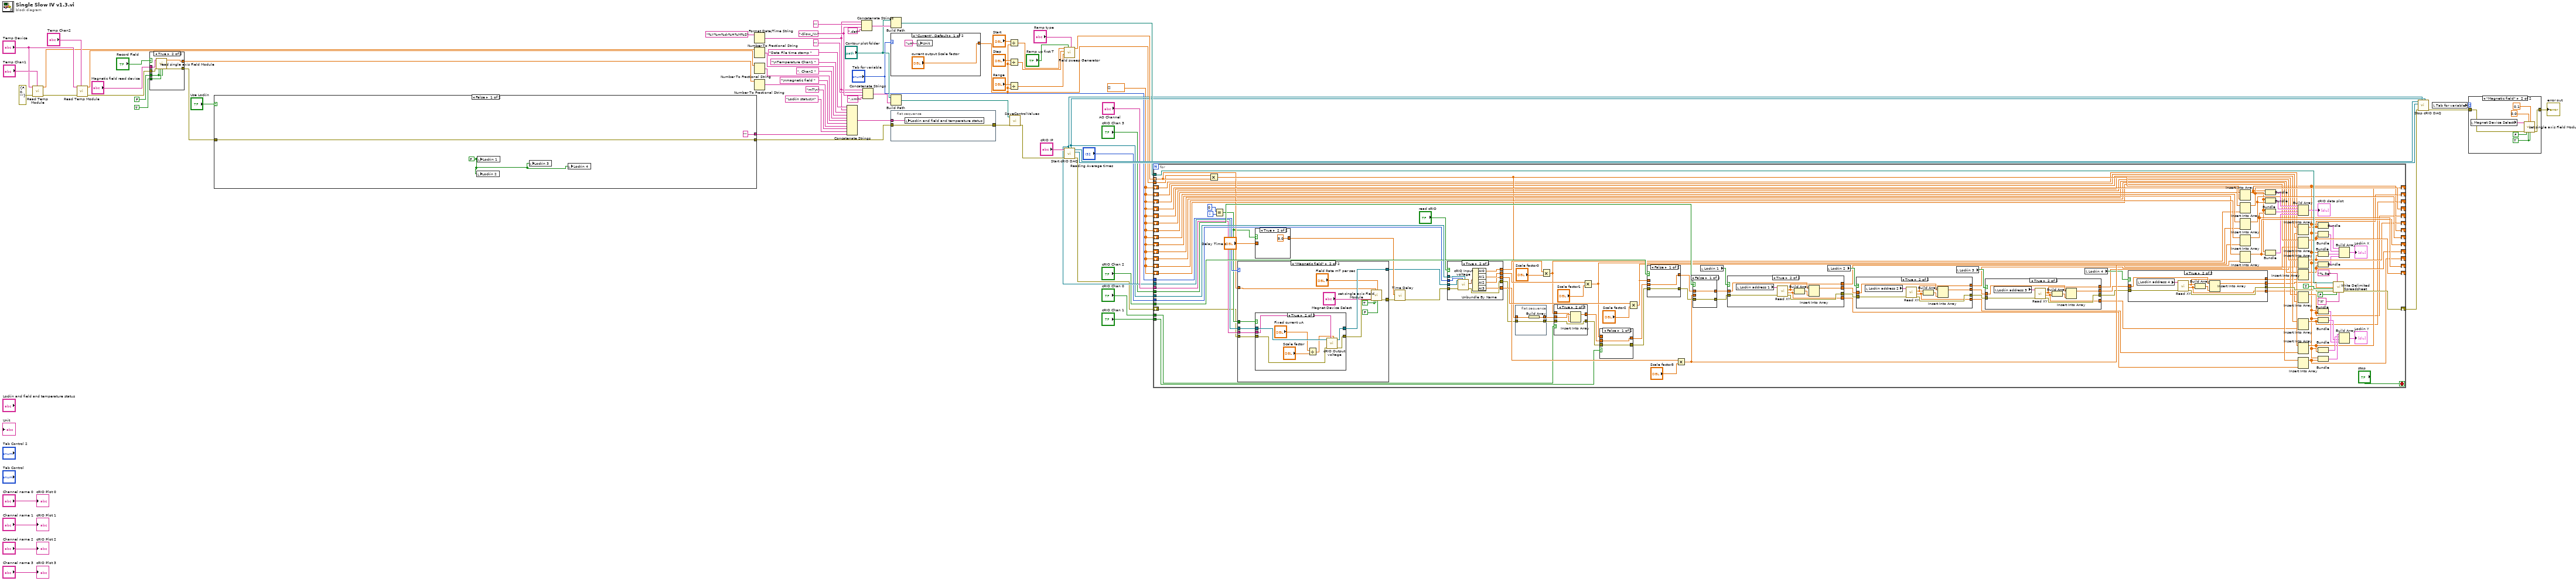
[diagram p0: block diagram]
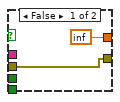
[diagram p2: hidden frame]
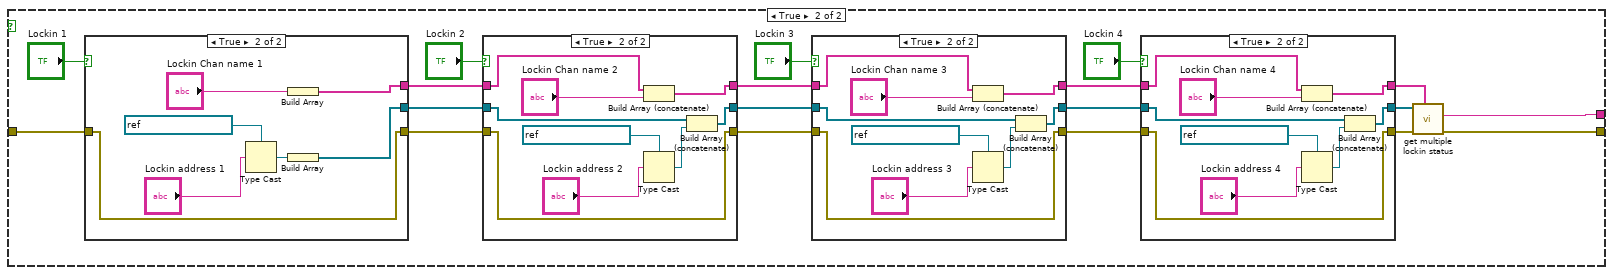
[diagram p3: hidden frame]
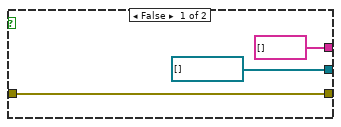
[diagram p7: hidden frame]
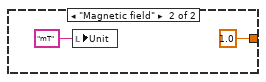
[diagram p9: hidden frame]
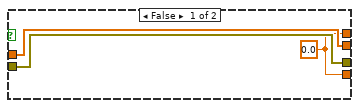
[diagram p10: hidden frame]
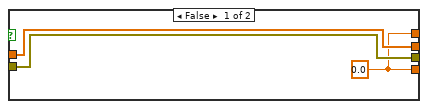
[diagram p11: hidden frame]
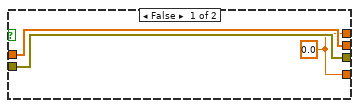
[diagram p12: hidden frame]
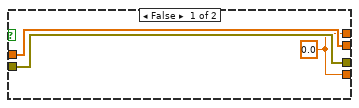
[diagram p13: hidden frame]
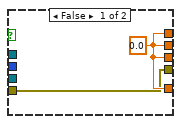
[diagram p15: hidden frame]
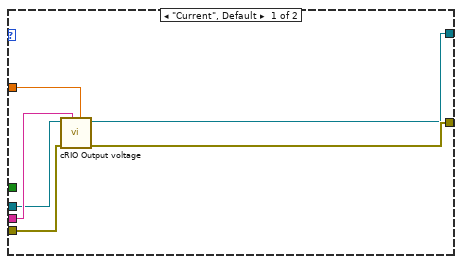
[diagram p16: hidden frame]
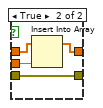
[diagram p19: hidden frame]
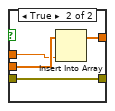
[diagram p20: hidden frame]
diagram:
  w2 = dbl[] []
  w67 = "-Slow_IV-"
  n1 = call "Read Temp Module.vi"("Temp Chan"="Temp Chan1", "error in (no error)"=errorcluster {"status"=FALSE, "code"=0, "source"=""} ("error in"), "Device"="Temp Device") -> ("error out"=w32:errorcluster, "Temperature K"=w27:dbl)  [unwired: 7 in]
  n2 = call "Read Temp Module.vi"("Temp Chan"="Temp Chan2", "error in (no error)"=w32, "Device"="Temp Device") -> ("error out"=w25:errorcluster, "Temperature K"=w26:dbl)  [unwired: 7 in]
  n3 = case shown="True" "Record Field" {
    tunnel: w25 -> [w75 w81]
    tunnel: "Magnetic field read device" -> [_ w80]
    tunnel: [inf w79] -> w23
    tunnel: TRUE ("Exec") -> [_ w78]
    tunnel: FALSE ("Init") -> [_ w77]
    tunnel: [w75 w76] -> w8
    frame False {
    }
    frame True {
      n4 = call "read single axis Field Module.vi"("Magnet Device Select"=w80, "error in (no error)"=w81, "Init"=w77, "Exec"=w78, "final"=w77) -> ("FIeld mT"=w79:dbl, "error out"=w76:errorcluster)  [unwired: 13 in]
    }
  }
  n5 = case shown="False" "Use Lockin" {
    tunnel: ["" ("Status output") w103] -> w9
    tunnel: [w84 w102] -> w7
    tunnel: w8 -> [w84 w97]
    frame False {
      w82 = FALSE ("Lockin 1")
      n6 = local write "Lockin 2"(w82) -> ()
      n7 = local write "Lockin 1"(w82) -> ()
      n8 = local write "Lockin 3"(w82) -> ()
      n9 = local write "Lockin 4"(w82) -> ()
    }
    frame True {
      n10 = case shown="True" "Lockin 1" {
        tunnel: w97 -> [w141 w149]
        tunnel: [w141 w149] -> w96
        tunnel: [refnum<visa-resource-name>[] [] w148] -> w92
        tunnel: [string[] [] w146] -> w88
        frame False {
        }
        frame True {
          n11 = Type Cast(type=refnum<visa-resource-name> "GPIB0::8::INSTR" ("Lockin address 1"), x="Lockin address 1") -> (*(type *) &x=w144:refnum<visa-resource-name>)
          n12 = Build Array("Lockin Chan name 1") -> (w146:string[])
          n13 = Build Array(w144) -> (w148:refnum<visa-resource-name>[])
        }
      }
      n14 = case shown="True" "Lockin 2" {
        tunnel: w96 -> [w129 w139]
        tunnel: [w129 w139] -> w95
        tunnel: w92 -> [w130 w138]
        tunnel: [w130 w137] -> w91
        tunnel: w88 -> [w128 w136]
        tunnel: [w128 w134] -> w87
        frame False {
        }
        frame True {
          n15 = Build Array (concatenate)(w136, "Lockin Chan name 2") -> (w134:string[])
          n16 = Type Cast(type=refnum<visa-resource-name> "GPIB0::8::INSTR" ("Lockin address 1"), x="Lockin address 2") -> (*(type *) &x=w132:refnum<visa-resource-name>)
          n17 = Build Array (concatenate)(w138, w132) -> (w137:refnum<visa-resource-name>[])
        }
      }
      n18 = case shown="True" "Lockin 3" {
        tunnel: w95 -> [w117 w127]
        tunnel: [w117 w127] -> w94
        tunnel: w91 -> [w118 w126]
        tunnel: [w118 w125] -> w90
        tunnel: w87 -> [w116 w123]
        tunnel: [w116 w122] -> w86
        frame False {
        }
        frame True {
          n19 = Build Array (concatenate)(w123, "Lockin Chan name 3") -> (w122:string[])
          n20 = Type Cast(type=refnum<visa-resource-name> "GPIB0::8::INSTR" ("Lockin address 1"), x="Lockin address 3") -> (*(type *) &x=w119:refnum<visa-resource-name>)
          n21 = Build Array (concatenate)(w126, w119) -> (w125:refnum<visa-resource-name>[])
        }
      }
      n22 = case shown="True" "Lockin 4" {
        tunnel: w94 -> [w105 w115]
        tunnel: [w105 w115] -> w93
        tunnel: w90 -> [w106 w114]
        tunnel: [w106 w113] -> w89
        tunnel: w86 -> [w104 w108]
        tunnel: [w104 w107] -> w85
        frame False {
        }
        frame True {
          n23 = Build Array (concatenate)(w108, "Lockin Chan name 4") -> (w107:string[])
          n24 = Type Cast(type=refnum<visa-resource-name> "GPIB0::8::INSTR" ("Lockin address 1"), x="Lockin address 4") -> (*(type *) &x=w111:refnum<visa-resource-name>)
          n25 = Build Array (concatenate)(w114, w111) -> (w113:refnum<visa-resource-name>[])
        }
      }
      n26 = call "get multiple lockin status.vi"("Device channel names"=w85, "error in (no error)"=w93, "SRS830 addresses"=w89) -> ("error out"=w102:errorcluster, "Status output"=w103:string)  [unwired: 6 in, 1 out]
    }
  }
  n27 = Format Date/Time String(time format string (%c)="%Y%m%d-%H%M%S") -> (date/time string=w19:string)  [unwired: 2 in]
  n28 = Number To Fractional String(number=w27) -> (F-format string=w16:string)  [unwired: 3 in]
  n29 = Number To Fractional String(number=w26) -> (F-format string=w15:string)  [unwired: 3 in]
  n30 = Number To Fractional String(number=w23) -> (F-format string=w13:string)  [unwired: 3 in]
  n31 = Concatenate Strings("Data File time stamp " ("string"), w19, "\nTemperature Chan1 " ("string"), w16, ", Chan2 " ("string"), w15, "\nmagnetic field " ("string"), w13, "mT\n" ("string"), "Lockin status\n" ("string"), w9) -> (w5:string)
  n32 = Concatenate Strings(w19, "" ("string"), w67, ".dat" ("string")) -> (w69:string)
  n33 = Concatenate Strings(w19, "" ("string"), w67, ".xml" ("string")) -> (w72:string)
  n34 = Build Path(base path="Contour plot folder", name or relative path=w69) -> (appended path=w52:path)
  n35 = case shown="\"Current\", Default" "Tab for variable" {
    tunnel: ["current output Scale factor" 1.0 ("current output Scale factor")] -> w36
    frame "Current", Default {
      n36 = local write "Unit"("uA" ("Unit")) -> ()
    }
    frame "Magnetic field" {
      n37 = local write "Unit"("mT" ("Unit")) -> ()
    }
  }
  n38 = Build Path(base path="Contour plot folder", name or relative path=w72) -> (appended path=w70:path)
  n39 = flat-sequence {
    tunnel: w7 -> [w155]
    tunnel: [w155] -> w6
    tunnel: w5 -> [w154]
    frame #0 {
      n40 = local write "Lockin and field and temperature status"(w154) -> ()
    }
  }
  n41 = Divide(x="Start", y=w36) -> (x/y=w38:dbl)
  n42 = Divide(x="Step", y=w36) -> (x/y=w56:dbl)
  n43 = Divide(x="Range", y=w36) -> (x/y=w55:dbl)
  n44 = call "SaveControlValues.vi"("XML File Path"=w70, "error in (no error)"=w6) -> ("error out"=w65:errorcluster)  [unwired: 8 in]
  n45 = call "Field sweep Generator.vi"("Ramp type"="Ramp type", "Ramp up first T"="Ramp up first T", "Field Radius"=w55, "Field step"=w56, "Field Origin"=w38) -> ("output array"=w53:dbl[])  [unwired: 6 in]
  n46 = call "Start cRIO DAQ.vi"("error in (no error)"=w65, "cRIO IP"="cRIO IP") -> ("error out"=w3:errorcluster, "vi reference"=w63:refnum<vi>, "application reference"=w64:refnum<vi>, "DAQ_AI_Reader endpoint"=w50:refnum<k21>, "DAQ_CMD_Writer endpoint"=w51:refnum<k21>)  [unwired: 5 in]
  n47 = for {
    tunnel: w51 -> [w226]
    tunnel: "AO Channel" -> [w227]
    tunnel: w53 -> [w228] mode=indexing
    tunnel: w50 -> [w268]
    tunnel: w52 -> [w267]
    tunnel: "cRIO Chan 1" -> [w253]
    tunnel: "cRIO Chan 2" -> [w252]
    tunnel: "cRIO Chan 3" -> [w251]
    shift-right: [w213] -> _
    shift-left: w2 -> [w244]
    shift-right: [w211] -> _
    shift-left: w2 -> [w243]
    shift-right: [w210] -> _
    shift-left: w2 -> [w242]
    shift-right: [w209] -> _
    shift-left: w2 -> [w241]
    shift-right: [w165] -> _
    shift-left: w2 -> [w237]
    tunnel: "Reading Average times" -> [w235]
    tunnel: "Tab for variable" -> [w229]
    tunnel: w36 -> [w222]
    tunnel: "cRIO Chan 0" -> [w220]
    shift-right: [w245] -> w44
    shift-left: w3 -> [w214]
    shift-right: [w194] -> _
    shift-left: w2 -> [w197]
    shift-right: [w193] -> _
    shift-left: w2 -> [w198]
    shift-right: [w192] -> _
    shift-left: w2 -> [w196]
    shift-right: [w191] -> _
    shift-left: w2 -> [w195]
    shift-right: [w169] -> _
    shift-left: w2 -> [w173]
    shift-right: [w168] -> _
    shift-left: w2 -> [w172]
    shift-right: [w167] -> _
    shift-left: w2 -> [w171]
    shift-right: [w166] -> _
    shift-left: w2 -> [w170]
    i -> [w233]
    stop <- "stop" stop-if-true
    n48 = Multiply(x=w222, y=w228) -> (x*y=w236:dbl)
    n49 = Equal?(x=0, y=w233) -> (x = y?=w223:bool)
    n50 = case shown="\"Magnetic field\"" w229 {
      tunnel: w228 -> [w336 w340]
      tunnel: w227 -> [w335 w344]
      tunnel: w214 -> [w334 w347]
      tunnel: w226 -> [w333 w346]
      tunnel: [w332 w342] -> w225
      tunnel: [w331 w345] -> w224
      tunnel: w223 -> [_ w348]
      frame "Current", Default {
        n51 = call "cRIO Output voltage.vi"("Voltage"=w336, "AO Channel"=w335, "error in (no error)"=w334, "DAQ_CMD_Writer endpoint"=w333) -> ("error out"=w332:errorcluster, "DAQ_CMD_Writer endpoint out"=w331:refnum<k21>)  [unwired: 6 in]
      }
      frame "Magnetic field" {
        w338 = TRUE ("Init")
        n52 = case shown="True" w348 {
          tunnel: w347 -> [w349 w358]
          tunnel: [w349 w357] -> w343
          tunnel: w346 -> [w350 w356]
          tunnel: [w350 w355] -> w345
          tunnel: w344 -> [_ w354]
          frame False {
          }
          frame True {
            n53 = Divide(x="Fixed current uA", y="Scale factor") -> (x/y=w352:dbl)
            n54 = call "cRIO Output voltage.vi"("Voltage"=w352, "AO Channel"=w354, "error in (no error)"=w358, "DAQ_CMD_Writer endpoint"=w356) -> ("error out"=w357:errorcluster, "DAQ_CMD_Writer endpoint out"=w355:refnum<k21>)  [unwired: 6 in]
          }
        }
        n55 = call "set single axis Field Module.vi"("Magnet Device Select"="Magnet Device Select", "error in (no error)"=w343, "Init"=w338, "Field Target mT"=w340, "Exec"=w338, "Field Rate mT per sec"="Field Rate mT per sec", "final"=FALSE ("Exec")) -> ("error out"=w342:errorcluster)  [unwired: 12 in]
      }
    }
    n56 = case shown="True" w223 {
      tunnel: "Delay Time s" -> [w359 _]
      tunnel: [w359 5.0 ("Delay Time s")] -> w230
      frame False {
      }
      frame True {
      }
    }
    n57 = call "Time Delay"("error in (no error)"=w225, "Delay Time (s)"=w230) -> ("error out"=w263:errorcluster)  [unwired: 9 in]
    n58 = case shown="True" "read cRIO" {
      tunnel: w268 -> [_ w330]
      tunnel: w263 -> [w319 w329]
      tunnel: [w320 w327] -> w262
      tunnel: [w320 w326] -> w261
      tunnel: [w320 w325] -> w260
      tunnel: [w320 w324] -> w259
      tunnel: [w319 w323] -> w248
      tunnel: w235 -> [_ w322]
      tunnel: w224 -> [_ w321]
      frame False {
        w320 = 0.0 ("AI2")
      }
      frame True {
        n59 = call "cRIO Input voltage.vi"("DAQ_AI_Reader endpoint"=w330, "Average"=w322, "error in (no error)"=w329, "DAQ_CMD_Writer endpoint"=w321) -> ("error out"=w323:errorcluster, "output cluster"=w328:T1)  [unwired: 5 in, 1 out]
        n60 = Unbundle By Name(w328) -> ("AI0"=w327:dbl, "AI1"=w326:dbl, "AI2"=w325:dbl, "AI3"=w324:dbl)
      }
    }
    n61 = flat-sequence {
      tunnel: w248 -> [w363]
      tunnel: [w363] -> w217
      tunnel: [w362] -> w219
      tunnel: w236 -> [w361]
      frame #0 {
        n62 = Build Array(w361) -> (w362:dbl[])
      }
    }
    n63 = Multiply(x=w262, y="Scale factor0") -> (x*y=w218:dbl)
    n64 = case shown="True" w220 {
      tunnel: w217 -> [w313 w318]
      tunnel: [w313 w318] -> w216
      tunnel: w219 -> [w314 w317]
      tunnel: w218 -> [_ w316]
      tunnel: [w314 w315] -> w215
      frame False {
      }
      frame True {
        n65 = Insert Into Array(array=w317, new element=w316) -> (w315:dbl[])  [unwired: 1 in]
      }
    }
    n66 = Multiply(x=w261, y="Scale factor1") -> (x*y=w240:dbl)
    n67 = case shown="False" w253 {
      tunnel: w216 -> [w376 w381]
      tunnel: [w376 w381] -> w250
      tunnel: w215 -> [w377 w380]
      tunnel: w240 -> [_ w379]
      tunnel: [w377 w378] -> w247
      frame False {
      }
      frame True {
        n68 = Insert Into Array(array=w380, new element=w379) -> (w378:dbl[])  [unwired: 1 in]
      }
    }
    n69 = Multiply(x=w260, y="Scale factor2") -> (x*y=w239:dbl)
    n70 = case shown="False" w252 {
      tunnel: w250 -> [w370 w375]
      tunnel: [w370 w375] -> w249
      tunnel: w247 -> [w371 w374]
      tunnel: w239 -> [_ w373]
      tunnel: [w371 w372] -> w246
      frame False {
      }
      frame True {
        n71 = Insert Into Array(array=w374, new element=w373) -> (w372:dbl[])  [unwired: 1 in]
      }
    }
    n72 = Multiply(x=w259, y="Scale factor3") -> (x*y=w238:dbl)
    n73 = case shown="False" w251 {
      tunnel: w249 -> [w364 w366]
      tunnel: w246 -> [w365 w369]
      tunnel: w238 -> [_ w368]
      tunnel: [w365 w367] -> w179
      tunnel: [w364 w366] -> w190
      frame False {
      }
      frame True {
        n74 = Insert Into Array(array=w369, new element=w368) -> (w367:dbl[])  [unwired: 1 in]
      }
    }
    n75 = local read "Lockin 1"() -> (w183:bool)
    n76 = case shown="True" w183 {
      tunnel: w190 -> [w270 w276]
      tunnel: [w270 w275] -> w203
      tunnel: w179 -> [w271 w278]
      tunnel: [w271 w279] -> w204
      tunnel: [w269 w273] -> w164
      tunnel: [w269 w272] -> w163
      frame False {
        w269 = 0.0 ("Y mV")
      }
      frame True {
        n77 = local read "Lockin address 1"() -> (w277:string)
        n78 = call "Read XY.vi"("error in (no error)"=w276, "VISA resource name"=w277) -> ("error out"=w275:errorcluster, "Y mV"=w272:dbl, "X mV"=w273:dbl)  [unwired: 6 in, 1 out]
        n79 = Build Array(w273, w272) -> (w274:dbl[])
        n80 = Insert Into Array(array=w278, new element=w274) -> (w279:dbl[])  [unwired: 1 in]
      }
    }
    n81 = local read "Lockin 2"() -> (w182:bool)
    n82 = case shown="True" w182 {
      tunnel: w203 -> [w303 w310]
      tunnel: [w303 w309] -> w199
      tunnel: w204 -> [w304 w307]
      tunnel: [w304 w308] -> w201
      tunnel: [w302 w306] -> w162
      tunnel: [w302 w305] -> w161
      frame False {
        w302 = 0.0 ("Y mV")
      }
      frame True {
        n83 = local read "Lockin address 2"() -> (w311:string)
        n84 = call "Read XY.vi"("error in (no error)"=w310, "VISA resource name"=w311) -> ("error out"=w309:errorcluster, "Y mV"=w305:dbl, "X mV"=w306:dbl)  [unwired: 6 in, 1 out]
        n85 = Build Array(w306, w305) -> (w312:dbl[])
        n86 = Insert Into Array(array=w307, new element=w312) -> (w308:dbl[])  [unwired: 1 in]
      }
    }
    n87 = local read "Lockin 3"() -> (w181:bool)
    n88 = case shown="True" w181 {
      tunnel: w199 -> [w292 w299]
      tunnel: [w292 w296] -> w200
      tunnel: w201 -> [w293 w298]
      tunnel: [w293 w297] -> w202
      tunnel: [w291 w295] -> w160
      tunnel: [w291 w294] -> w159
      frame False {
        w291 = 0.0 ("X mV")
      }
      frame True {
        n89 = local read "Lockin address 3"() -> (w300:string)
        n90 = call "Read XY.vi"("error in (no error)"=w299, "VISA resource name"=w300) -> ("error out"=w296:errorcluster, "Y mV"=w294:dbl, "X mV"=w295:dbl)  [unwired: 6 in, 1 out]
        n91 = Build Array(w295, w294) -> (w301:dbl[])
        n92 = Insert Into Array(array=w298, new element=w301) -> (w297:dbl[])  [unwired: 1 in]
      }
    }
    n93 = local read "Lockin 4"() -> (w180:bool)
    n94 = case shown="True" w180 {
      tunnel: w200 -> [w281 w288]
      tunnel: w202 -> [w282 w285]
      tunnel: [w282 w286] -> w156
      tunnel: [w281 w287] -> w189
      tunnel: [w280 w284] -> w158
      tunnel: [w280 w283] -> w157
      frame False {
        w280 = 0.0 ("X mV")
      }
      frame True {
        n95 = local read "Lockin address 4"() -> (w289:string)
        n96 = call "Read XY.vi"("error in (no error)"=w288, "VISA resource name"=w289) -> ("error out"=w287:errorcluster, "Y mV"=w283:dbl, "X mV"=w284:dbl)  [unwired: 6 in, 1 out]
        n97 = Build Array(w284, w283) -> (w290:dbl[])
        n98 = Insert Into Array(array=w285, new element=w290) -> (w286:dbl[])  [unwired: 1 in]
      }
    }
    n99 = Insert Into Array(array=w237, new element=w236) -> (w165:dbl[])  [unwired: 1 in]
    n100 = Insert Into Array(array=w244, new element=w218) -> (w213:dbl[])  [unwired: 1 in]
    n101 = Insert Into Array(array=w243, new element=w240) -> (w211:dbl[])  [unwired: 1 in]
    n102 = Insert Into Array(array=w242, new element=w239) -> (w210:dbl[])  [unwired: 1 in]
    n103 = Insert Into Array(array=w241, new element=w238) -> (w209:dbl[])  [unwired: 1 in]
    n104 = Bundle(w165, w213) -> (w212:cluster{dbl[], dbl[]})  [unwired: 1 in]
    n105 = Bundle(w165, w211) -> (w208:cluster{dbl[], dbl[]})  [unwired: 1 in]
    n106 = Bundle(w165, w210) -> (w207:cluster{dbl[], dbl[]})  [unwired: 1 in]
    n107 = Bundle(w165, w209) -> (w206:cluster{dbl[], dbl[]})  [unwired: 1 in]
    n108 = Build Array(w212, w208, w207, w206) -> (→"cRIO data plot":cluster{dbl[], dbl[]}[])
    n109 = Insert Into Array(array=w197, new element=w164) -> (w194:dbl[])  [unwired: 1 in]
    n110 = Insert Into Array(array=w198, new element=w162) -> (w193:dbl[])  [unwired: 1 in]
    n111 = Insert Into Array(array=w196, new element=w160) -> (w192:dbl[])  [unwired: 1 in]
    n112 = Insert Into Array(array=w195, new element=w158) -> (w191:dbl[])  [unwired: 1 in]
    n113 = Insert Into Array(array=w170, new element=w157) -> (w166:dbl[])  [unwired: 1 in]
    n114 = Insert Into Array(array=w171, new element=w159) -> (w167:dbl[])  [unwired: 1 in]
    n115 = Insert Into Array(array=w172, new element=w161) -> (w168:dbl[])  [unwired: 1 in]
    n116 = Insert Into Array(array=w173, new element=w163) -> (w169:dbl[])  [unwired: 1 in]
    n117 = Bundle(w165, w194) -> (w188:cluster{dbl[], dbl[]})  [unwired: 1 in]
    n118 = Bundle(w165, w193) -> (w187:cluster{dbl[], dbl[]})  [unwired: 1 in]
    n119 = Bundle(w165, w192) -> (w186:cluster{dbl[], dbl[]})  [unwired: 1 in]
    n120 = Bundle(w165, w191) -> (w185:cluster{dbl[], dbl[]})  [unwired: 1 in]
    n121 = Bundle(w165, w166) -> (w175:cluster{dbl[], dbl[]})  [unwired: 1 in]
    n122 = Bundle(w165, w167) -> (w176:cluster{dbl[], dbl[]})  [unwired: 1 in]
    n123 = Bundle(w165, w168) -> (w177:cluster{dbl[], dbl[]})  [unwired: 1 in]
    n124 = Bundle(w165, w169) -> (w178:cluster{dbl[], dbl[]})  [unwired: 1 in]
    n125 = call-poly <vilib>:"Write Delimited Spreadsheet.vi"("file path (dialog if empty)"=w267, "format (%.3f)"="%.9e", "1D data"=w156, "append to file? (new file:F)"=TRUE, "error in (no error)"=w189, "transpose? (no:F)"=FALSE, "delimiter (\\t)"="\t" ("delimiter (\\t)")) -> ("error out"=w245:errorcluster)  [unwired: 7 in, 1 out]
    n126 = Build Array(w188, w187, w186, w185) -> (→"Lockin X":cluster{dbl[], dbl[]}[])
    n127 = Build Array(w178, w177, w176, w175) -> (→"Lockin Y":cluster{dbl[], dbl[]}[])
  }
  n128 = call "Stop cRIO DAQ.vi"("DAQ_AI_Reader endpoint"=w50, "DAQ_CMD_Writer endpoint"=w51, "error in (no error)"=w44, "VI reference"=w63, "application reference"=w64) -> ("error out"=w34:errorcluster)  [unwired: 6 in]
  n129 = local read "Tab for variable"() -> (w35:enum32{"Current", "Magnetic field"})
  n130 = case shown="\"Magnetic field\"" w35 {
    tunnel: w34 -> [w382 w386]
    tunnel: [w382 w385] -> w33
    frame "Current", Default {
    }
    frame "Magnetic field" {
      w383 = TRUE ("Exec")
      n131 = local read "Magnet Device Select"() -> (w389:string)
      n132 = call "set single axis Field Module.vi"("Magnet Device Select"=w389, "error in (no error)"=w386, "Init"=FALSE, "Field Target mT"=0.0, "Exec"=w383, "Field Rate mT per sec"=0.1, "final"=w383) -> ("error out"=w385:errorcluster)  [unwired: 12 in]
    }
  }
  "error out" <- w33
  "cRIO Plot 0" <- "Channel name 0"
  "cRIO Plot 1" <- "Channel name 1"
  "cRIO Plot 2" <- "Channel name 2"
  "cRIO Plot 3" <- "Channel name 3"
